vi "Keyence ActiveX TimeOut.vi"(8 "error in (no error)":errorcluster, 10 "Status in":T1, 11 "Automation Refnum in":refnum<k7>) -> (0 "error out":errorcluster, 2 "Status out":T1)   [LabVIEW 2014]
uses:
  Keyence Status.ctl
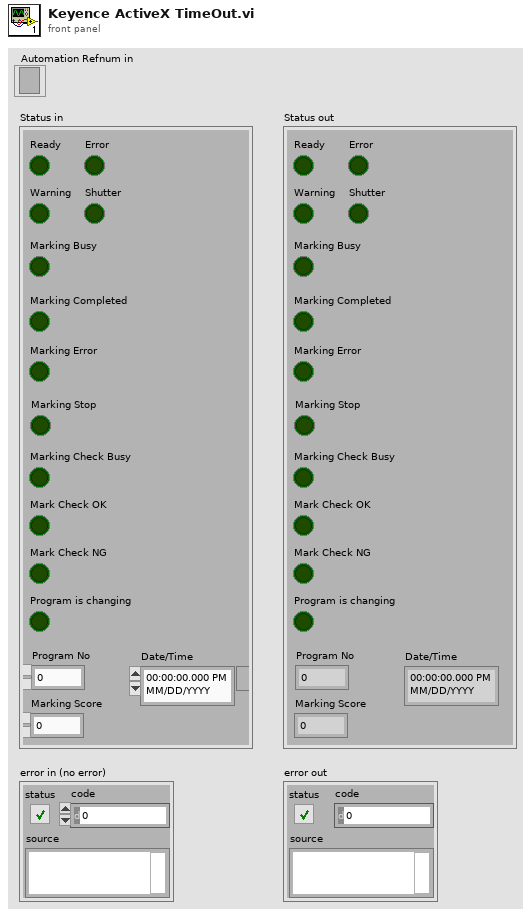
[diagram p1: front panel]
types:
  T1 = typedef "Keyence Status.ctl" = cluster{"Ready":bool, "Error":bool, "Warning":bool, "Shutter":bool, "Mark Check OK":bool, "Mark Check NG":bool, "Marking Busy":bool, "Program No":u16, "Marking Check Busy":bool, "Marking Completed":bool, "Marking Score":u16, "Marking Error":bool, "Marking Stop":bool, "Program is changing":bool, "Date/Time":timestamp}
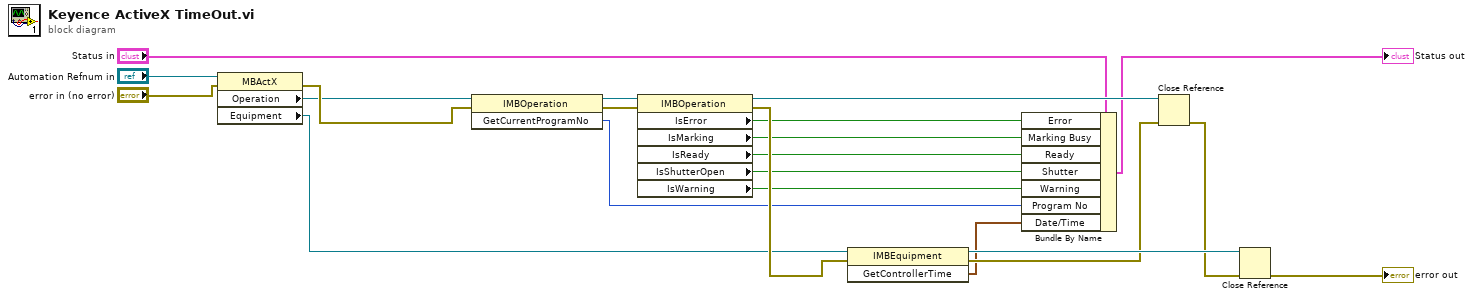
[diagram p0: block diagram]
diagram:
  n1 = property class="MBActX"(reference="Automation Refnum in", error in="error in (no error)") -> (error out=w20:errorcluster, "Operation"=w15:refnum<k7>, "Equipment"=w18:refnum<k7>)  [unwired: 1 out]
  n2 = invoke class="IMBOperation" method="GetCurrentProgramNo"(reference=w15, error in=w20) -> (reference out=w16:refnum<k7>, error out=w14:errorcluster, "GetCurrentProgramNo"=w2:i32)  [unwired: 1 in]
  n3 = property class="IMBOperation"(reference=w16, error in=w14) -> (reference out=w17:refnum<k7>, error out=w21:errorcluster, "IsError"=w9:bool, "IsMarking"=w10:bool, "IsReady"=w11:bool, "IsShutterOpen"=w12:bool, "IsWarning"=w13:bool)
  n4 = invoke class="IMBEquipment" method="GetControllerTime"(reference=w18, error in=w21) -> (reference out=w19:refnum<k7>, error out=w4:errorcluster, "GetControllerTime"=w3:timestamp)  [unwired: 1 in]
  n5 = Bundle By Name(cluster="Status in", "Error"=w9, "Marking Busy"=w10, "Ready"=w11, "Shutter"=w12, "Warning"=w13, "Program No"=w2, "Date/Time"=w3) -> (→"Status out":T1)
  n6 = Close Reference(reference=w17, error in (no error)=w4) -> (error out=w1:errorcluster)
  n7 = Close Reference(reference=w19, error in (no error)=w1) -> (error out=→"error out":errorcluster)
